vi "SP Prepare for Downloading Stimulus.vi"(5 "Current Stimulus":T1={"Use Instrument Settings"=FALSE, "Blank Frequencies"=FALSE, "Sweep Type"=enum."Linear", "Sweep"={"Fstart"=500.0, "Fstop"=1500.0, "Units"=enum."MHz", "Points"=201}, "Power (dBm)"=999.0, "IFBW (Hz)"=-1.0, "Sweep Time (s)"=-1.0, "Calibration"={"State"=FALSE, "String"=""}} {"Sweep Time (s)" format="%.3g"}, 7 "Requested Stimulus":T1={"Use Instrument Settings"=FALSE, "Blank Frequencies"=FALSE, "Sweep Type"=enum."Linear", "Sweep"={"Fstart"=500.0, "Fstop"=1500.0, "Units"=enum."MHz", "Points"=201}, "Power (dBm)"=999.0, "IFBW (Hz)"=-1.0, "Sweep Time (s)"=-1.0, "Calibration"={"State"=FALSE, "String"=""}} {"Sweep Time (s)" format="%.3g"}, 8 "error in (no error)":errorcluster, 9 "Stimulus Changing? (f)":bool, 10 "Parameters to Measure":T4[](array[typedef]) {"Channel" min=1 max=99 step=1; "Parameter"."Stimulus Port" min=1 step=1; "Parameter"."Response Port" min=1 step=1}, 11 "Currnet Parameters to Measure":T4[](array[typedef]) {"Channel" min=1 max=99 step=1; "Parameter"."Stimulus Port" min=1 step=1; "Parameter"."Response Port" min=1 step=1}) -> (0 "error out":errorcluster, 3 "Action":T7)   [LabVIEW 2011]
uses:
  TypeDefs/SP Dialog Response.ctl
  TypeDefs/SP Parameter to Measure.ctl
  TypeDefs/SP Parameter.ctl
  TypeDefs/SP Calibration State.ctl
  TypeDefs/SP Measurement Format.ctl
  TypeDefs/SP Stimulus Parameters.ctl
  TypeDefs/SP Frequency Units.ctl
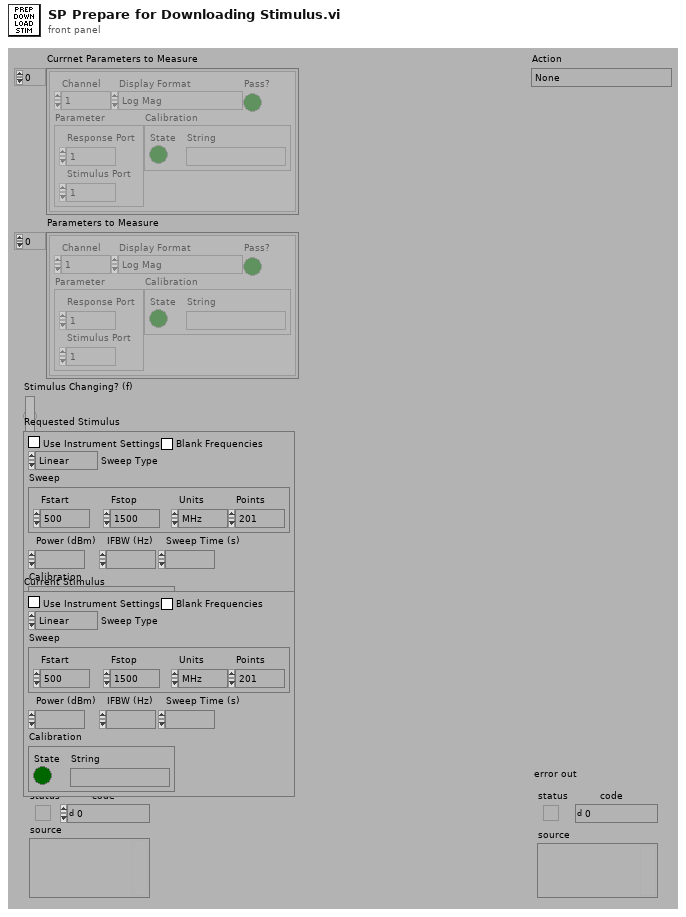
[diagram p1: front panel]
types:
  T1 = typedef "SP Stimulus Parameters.ctl" = cluster{"Use Instrument Settings":bool, "Blank Frequencies":bool, "Sweep Type":enum32{"Linear", "Logarithmic", "List", "Power", "CW"}, "Sweep":cluster{"Fstart":dbl, "Fstop":dbl, "Units":T2, "Points":i32}, "Power (dBm)":dbl, "IFBW (Hz)":dbl, "Sweep Time (s)":dbl, "Calibration":T3}
  T2 = typedef "SP Frequency Units.ctl" = enum16{"Hz", "kHz", "MHz", "GHz", "Points"}
  T3 = typedef "SP Calibration State.ctl" = cluster{"State":bool, "String":string}
  T4 = typedef "SP Parameter to Measure.ctl" = cluster{"Channel":i8, "Parameter":T5, "Calibration":T3, "Display Format":T6, "Pass?":bool}
  T5 = typedef "SP Parameter.ctl" = cluster{"Stimulus Port":i8, "Response Port":i8}
  T6 = typedef "SP Measurement Format.ctl" = enum32{"Log Mag", "Phase", "Delay", "Smith (R+jX)", "Polar (Re/Im)", "Linear Mag", "SWR", "Real", "Imaginary", "Smith (Lin/Phase)", "Smith (Log/Phase)", "Smith (Real/Imag)", "Smith (G+jB)", "Polar (Lin/Phase)", "Polar (Log/Phase)", "Expanded Phase", "Positive Phase", "Inverted Smith", "Unwrapped Phase", "Power Out", "Power In", "Linear Mag/Phase", "Log Mag/Phase", "Real/Imaginary"}
  T7 = typedef "SP Dialog Response.ctl" = enum16{"None", "Calibrate", "Restore", "Ignore", "Abort", "Abort All"}
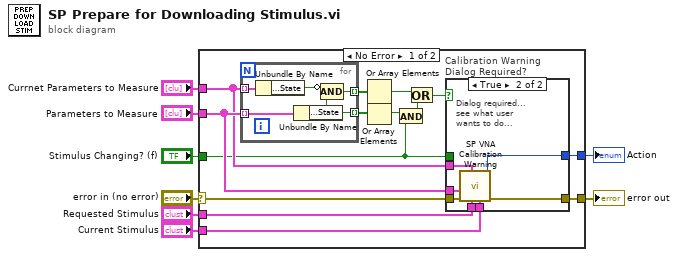
[diagram p0: block diagram]
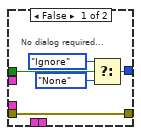
[diagram p2: hidden frame]
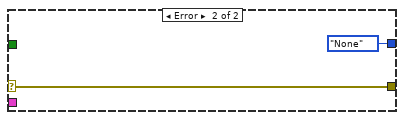
[diagram p3: hidden frame]
diagram:
  n1 = case shown="No Error" "error in (no error)" {
    selector: "error in (no error)" -> [w9 w41]
    tunnel: "Parameters to Measure" -> [w21 _]
    tunnel: "Currnet Parameters to Measure" -> [w20 _]
    tunnel: "Requested Stimulus" -> [w19 _]
    tunnel: "Current Stimulus" -> [w18 _]
    tunnel: [w17 w41] -> w4
    tunnel: [w16 SP_Dialog_Response."None" ("Choice")] -> w3
    tunnel: "Stimulus Changing? (f)" -> [w11 _]
    frame No Error {
      n2 = for {
        tunnel: w20 -> [w36] mode=indexing
        tunnel: [w38] -> w22 mode=indexing
        tunnel: w21 -> [w39] mode=indexing
        tunnel: [w37] -> w15 mode=indexing
        n3 = Unbundle By Name(w36) -> ("Calibration.State"=w35:bool)
        n4 = Unbundle By Name(w39) -> ("Calibration.State"=w37:bool)
        n5 = Compound Arithmetic op=AND(invert w35, w37) -> (w38:bool)
      }
      n6 = Or Array Elements(Boolean array=w22) -> (logical OR=w14:bool)
      n7 = Or Array Elements(Boolean array=w15) -> (logical OR=w12:bool)
      n8 = And(x=w12, y=w11) -> (x .and. y?=w10:bool)
      n9 = Or(x=w14, y=w10) -> (x .or. y?=w13:bool)
      n10 = case "Calibration Warning Dialog Required?" shown="True" w13 {
        tunnel: w9 -> [w27 w34]
        tunnel: [w27 w33] -> w17
        tunnel: [w25 w28] -> w16
        tunnel: w21 -> [_ w32]
        tunnel: w19 -> [_ w31]
        tunnel: w18 -> [_ w30]
        tunnel: w20 -> [_ w29]
        tunnel: w11 -> [w24 _]
        frame False {
          # "No dialog required..."
          n11 = Select(t=SP_Dialog_Response."Ignore" ("Action"), s=w24, f=SP_Dialog_Response."None" ("Action")) -> (s? t:f=w25:T7)
        }
        frame True {
          # "Dialog required...\nsee what user\nwants to do..."
          n12 = call "SP VNA Calibration Warning.vi"("Current Stimulus"=w30, "Requested Stimulus"=w31, "Current Parameters to Measure"=w29, "error in (no error)"=w34, "Parameters to Measure"=w32) -> ("error out"=w33:errorcluster, "Choice"=w28:T7)  [unwired: 2 in, 3 out]
        }
      }
    }
    frame Error {
    }
  }
  "error out" <- w4
  "Action" <- w3
